vi "LABVIEW_0416043-1.vi"() -> ()   [LabVIEW 2015]
uses:
  <vilib>/Analysis/2dsp.llb/Real FFT.vi
  <vilib>/Utility/file.llb/Read From Spreadsheet File (DBL).vi
  <vilib>/Analysis/NI_AALPro.lvlib
panel:
  out "amplitude":ext
  out "frequency":ext
  out "FFT {X}":dbl[][](graph)
  out "CSV file path":path
  out "Input1":dbl[](graph)
  # "1. ¶}±ÒÀÉ®×¡AÆ[¹îŠ‹xe®t²§¡C  (ÀÉ¦W:XXX.csv)"
  # "4. HTþsŠ‹xe„vFFT"
  # "3. iQŠ‹xeKNBfßWW"
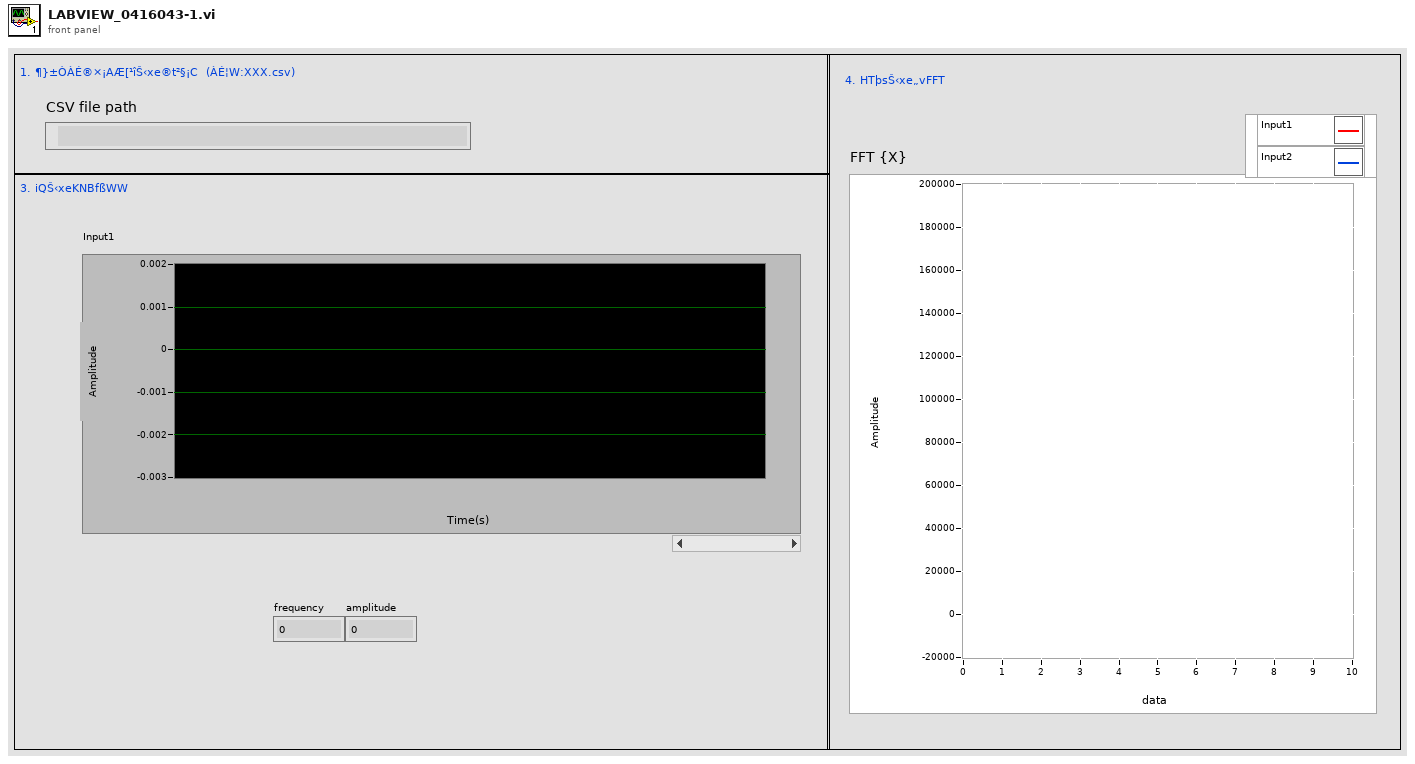
[diagram p1: front panel]
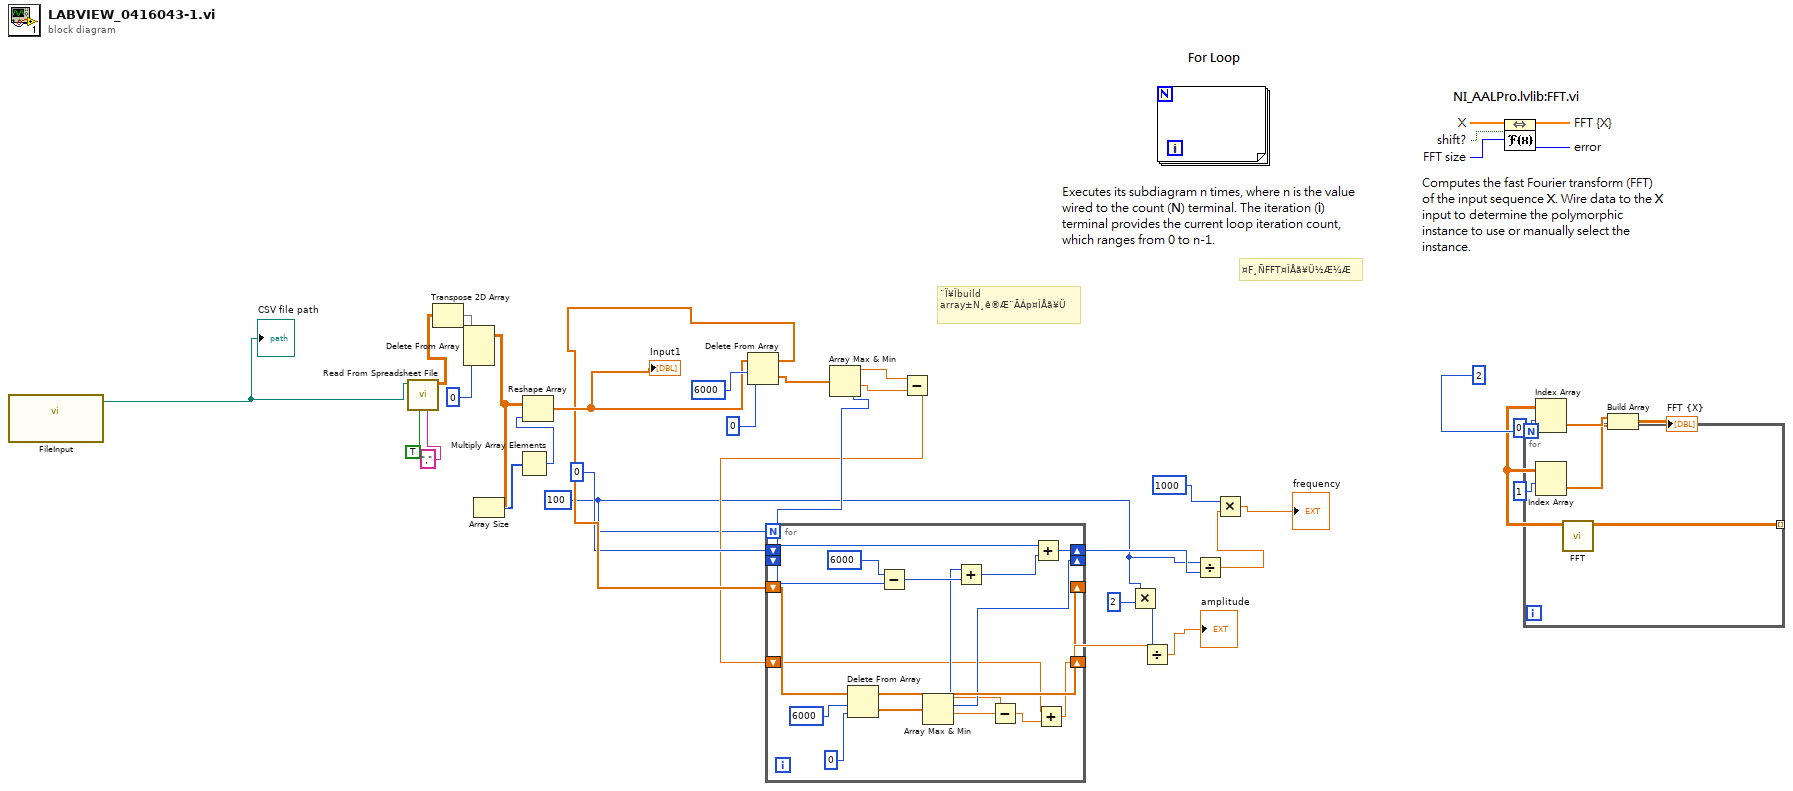
[diagram p0: block diagram]
diagram:
  w2 = 100
  # "了解FFT及顯示複數"
  # "使用build array將資料並聯及顯示"
  n1 = call "FileInput.vi"() -> ("Path"=w29:path)  [unwired: 18 in, 1 out]
  "CSV file path" <- w29
  n2 = call-poly <vilib>:"Read From Spreadsheet File.vi"("delimiter (\\t)"="," ("delimiter (\\t)"), "transpose (no:F)"=TRUE, "file path (dialog if empty)"=w29) -> ("all rows"=w23:dbl[][])  [unwired: 4 in, 4 out]
  n3 = Transpose 2D Array(2D array=w23) -> (transposed array=w22:dbl[][])
  n4 = Delete From Array(array=w22, index (col)=0) -> (array with subset deleted=w26:dbl[][])  [unwired: 2 in, 1 out]
  n5 = Array Size(array=w26) -> (size(s)=w25:i32[])
  n6 = Multiply Array Elements(1:w25) -> (0:w24:i32)
  n7 = Reshape Array(w26, w24) -> (w17:dbl[])
  "Input1" <- w17
  n8 = Delete From Array(array=w17, length=6000, index=0) -> (deleted portion=w16:dbl[], array with subset deleted=w15:dbl[])
  n9 = Array Max & Min(array=w16) -> (max value=w9:dbl, max index (indices)=w14:i32, min value=w12:dbl)  [unwired: 1 out]
  n10 = Subtract(x=w9, y=w12) -> (x-y=w10:dbl)
  n11 = for {
    N: w2 -> [_]
    shift-right: [w48] -> _
    shift-left: w15 -> [w49]
    shift-right: [w41] -> _
    shift-left: w14 -> [w44]
    shift-right: [w47] -> w7
    shift-left: 0 -> [w46]
    shift-right: [w37] -> w11
    shift-left: w10 -> [w36]
    n12 = Delete From Array(array=w49, length=6000, index=0) -> (deleted portion=w50:dbl[], array with subset deleted=w48:dbl[])
    n13 = Subtract(x=6000, y=w44) -> (x-y=w43:i32)
    n14 = Array Max & Min(array=w50) -> (max value=w40:dbl, max index (indices)=w41:i32, min value=w39:dbl)  [unwired: 1 out]
    n15 = Add(x=w41, y=w43) -> (x+y=w42:i32)
    n16 = Subtract(x=w40, y=w39) -> (x-y=w38:dbl)
    n17 = Add(x=w46, y=w42) -> (x+y=w47:i32)
    n18 = Add(x=w36, y=w38) -> (x+y=w37:dbl)
  }
  n19 = Multiply(x=w2, y=2) -> (x*y=w1:i32)
  n20 = Divide(x=w11, y=w1) -> (x/y=→"amplitude":dbl)
  n21 = Divide(x=w2, y=w7) -> (x/y=w6:dbl)
  n22 = Multiply(x=1000, y=w6) -> (x*y=→"frequency":dbl)
  n23 = for {
    N: 2 -> [_]
    tunnel: [w53] -> w20 mode=indexing
    n24 = call-poly <vilib>:"FFT.vi"() -> ("FFT {X}"=w53:cdb[])  [unwired: 10 in, 1 out]
  }
  n25 = Index Array "Index Array"(array=w20, index (row)=0 ("disabled index (col)")) -> (element=w34:cdb[])  [unwired: 1 in]
  n26 = Index Array "Index Array"(array=w20, index (row)=1 ("disabled index (col)")) -> (element=w33:cdb[])  [unwired: 1 in]
  n27 = Build Array "Build Array"(w34, w33) -> (→"FFT {X}":cdb[][])
